vi "_Parse ACLR Segment Limit Check Result.vi"(8 "error in (no error)":errorcluster, 10 "Input String":string, 11 "VISA resource name":refnum<visa-resource-name>) -> (0 "error out":errorcluster, 1 "ACLR Limit Check Results":T2, 2 "Reliability Results":T1, 3 "VISA resource name out":refnum<visa-resource-name>, 5 "Out Of Tolerance":i32, 7 "Statistic Expired":i32)   [LabVIEW 2020, in "Rohde&Schwarz CMWXP NR FR1 Measurement.lvlib"]
uses:
  <instrlib>/Rohde&Schwarz CMWXP NR FR1 Measurement/Rohde&Schwarz CMWXP NR FR1 Measurement.lvlib
  <instrlib>/Rohde&Schwarz CMWXP NR FR1 Measurement/Private/_SegReliability.ctl
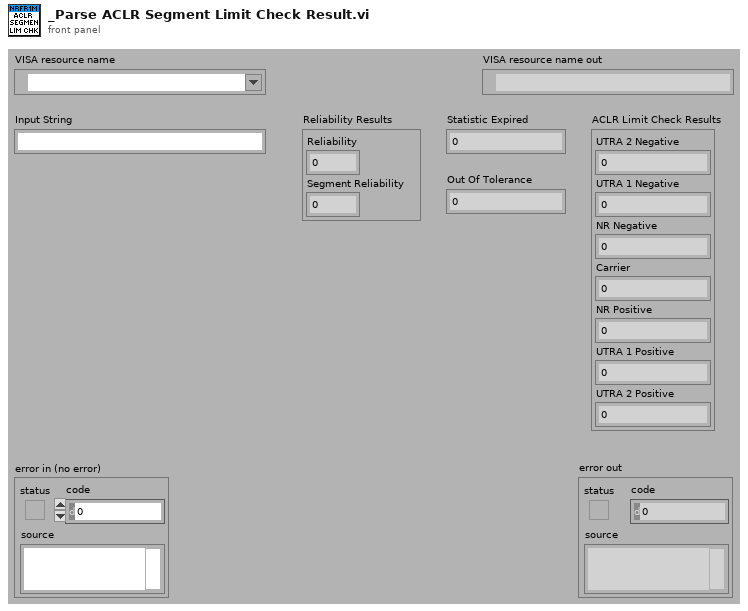
[diagram p1: front panel]
types:
  T1 = typedef "Rohde&Schwarz CMWXP NR FR1 Measurement.lvlib/_SegReliability.ctl" = cluster{"Reliability":i32, "Segment Reliability":i32}
  T2 = cluster{"UTRA 2 Negative":i32, "UTRA 1 Negative":i32, "NR Negative":i32, "Carrier":i32, "NR Positive":i32, "UTRA 1 Positive":i32, "UTRA 2 Positive":i32}
  T3 = cluster{"Limit Check Value":i32, "Limit Check Value":i32, "Limit Check Value":i32, "Limit Check Value":i32, "Limit Check Value":i32, "Limit Check Value":i32, "Limit Check Value":i32}
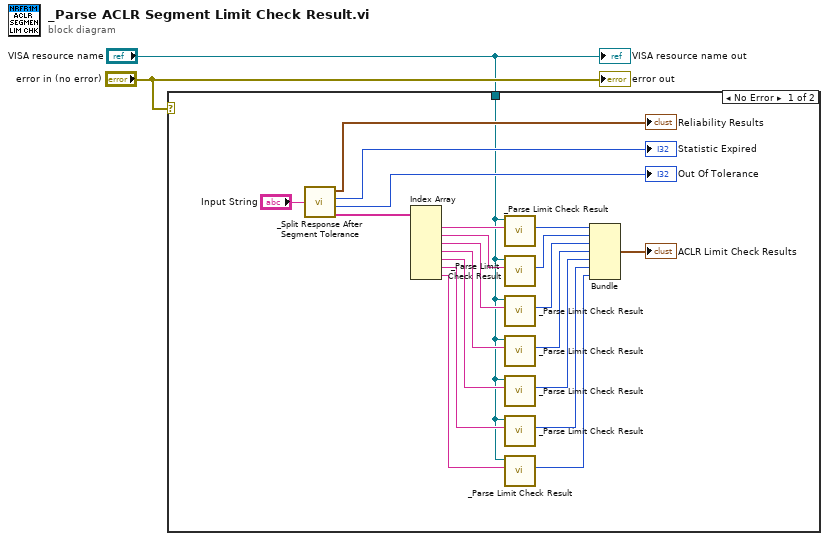
[diagram p0: block diagram]
diagram:
  n1 = case shown="No Error" "error in (no error)" {
    tunnel: "VISA resource name" -> [w3 _]
    frame No Error {
      n2 = call <instrlib>:"_Split Response After Segment Tolerance.vi"("Input String"="Input String") -> ("Reliability Results"=→"Reliability Results":T1, "Statistic Expired"=→"Statistic Expired":i32, "Out Of Tolerance"=→"Out Of Tolerance":i32, "Response out"=w5:string[])
      n3 = Index Array(array=w5) -> (element #1=w16:string, element #2=w15:string, element #3=w14:string, element #4=w10:string, element #5=w11:string, element #6=w12:string, element #7=w13:string)  [unwired: 7 in]
      n4 = call <instrlib>:"_Parse Limit Check Result.vi"("String Value In"=w16, "VISA resource name"=w3) -> ("Limit Check Value"=w19:i32)  [unwired: 7 in, 2 out]
      n5 = call <instrlib>:"_Parse Limit Check Result.vi"("String Value In"=w15, "VISA resource name"=w3) -> ("Limit Check Value"=w18:i32)  [unwired: 7 in, 2 out]
      n6 = call <instrlib>:"_Parse Limit Check Result.vi"("String Value In"=w14, "VISA resource name"=w3) -> ("Limit Check Value"=w17:i32)  [unwired: 7 in, 2 out]
      n7 = call <instrlib>:"_Parse Limit Check Result.vi"("String Value In"=w10, "VISA resource name"=w3) -> ("Limit Check Value"=w9:i32)  [unwired: 7 in, 2 out]
      n8 = call <instrlib>:"_Parse Limit Check Result.vi"("String Value In"=w11, "VISA resource name"=w3) -> ("Limit Check Value"=w8:i32)  [unwired: 7 in, 2 out]
      n9 = call <instrlib>:"_Parse Limit Check Result.vi"("String Value In"=w12, "VISA resource name"=w3) -> ("Limit Check Value"=w7:i32)  [unwired: 7 in, 2 out]
      n10 = call <instrlib>:"_Parse Limit Check Result.vi"("String Value In"=w13, "VISA resource name"=w3) -> ("Limit Check Value"=w6:i32)  [unwired: 7 in, 2 out]
      n11 = Bundle("Limit Check Value"=w19, "Limit Check Value"=w18, "Limit Check Value"=w17, "Limit Check Value"=w9, "Limit Check Value"=w8, "Limit Check Value"=w7, "Limit Check Value"=w6) -> (→"ACLR Limit Check Results":T3)  [unwired: 1 in]
    }
    frame Error {
    }
  }
  "error out" <- "error in (no error)"
  "VISA resource name out" <- "VISA resource name"
